vi "lsl get info.vi"(8 "error in (no error)":errorcluster, 11 "outlet":T2) -> (0 "error out":errorcluster, 3 "streaminfo":T1)   [LabVIEW 2016, in "Lab Streaming Layer.lvlib"]
doc: "extern LIBLSL_C_API lsl_streaminfo lsl_get_info(lsl_outlet out);"
uses:
  Lab Streaming Layer.lvlib
  liblsl-LabVIEW-master/liblsl-LabVIEW-master/lsl.dll
  Custom Controls/lsl_outlet.ctl
  Custom Controls/lsl_streaminfo.ctl
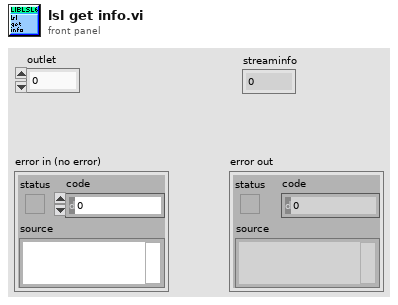
[diagram p1: front panel]
types:
  T1 = typedef "liblsl-LabVIEW.lvlib/lsl_streaminfo.ctl" = u64
  T2 = typedef "liblsl-LabVIEW.lvlib/lsl_outlet.ctl" = u64
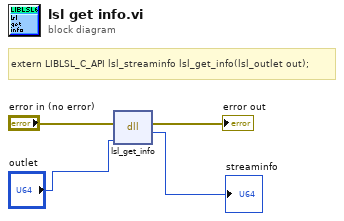
[diagram p0: block diagram]
diagram:
  # "extern LIBLSL_C_API lsl_streaminfo lsl_get_info(lsl_outlet out);"
  n1 = dll-call lib="E:/LabStreamingLayer/liblsl-LabVIEW-master/liblsl-LabVIEW-master/lsl.dll" fn="lsl_get_info"(error in="error in (no error)", "out"="outlet") -> (error out=→"error out":errorcluster, "return type"=→"streaminfo":u64)  [unwired: 3 in, 1 out]
